vi "Read Self Attributes.vi"(11 "Teller in":refnum<class "Teller.lvclass">) -> (2 "Self Attributes":refnum<class "Attributes.lvclass">)   [LabVIEW 2025, in "jettl.lvlib" / "Teller.lvlib" / "Teller.lvclass"]
uses:
  Teller.lvclass
  Attributes/Attributes/Attributes.lvclass
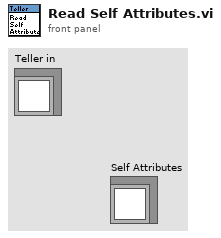
[diagram p1: front panel]
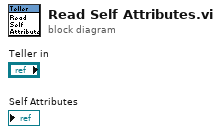
[diagram p0: block diagram]
diagram:
